vi "CL3IF_GetProgramNo.vi"(8 "error in":errorcluster {"code" format="%x"}, 11 "deviceId":i32) -> (0 "error out":errorcluster {"code" format="%x"}, 2 "programNo":u8)   [LabVIEW 2020, in "Keyence CL-3000.lvlib"]
doc: "This function gets the current program number."
uses:
  Keyence CL-3000.lvlib
  Private/enums/Function Name.ctl
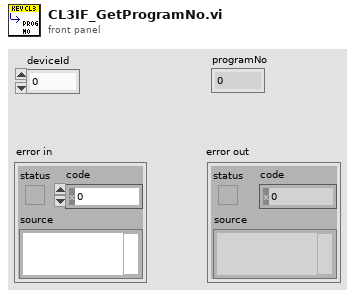
[diagram p1: front panel]
types:
  T1 = typedef "Keyence CL-3000.lvlib/Function Name.ctl" = enum16{"Initialize", "Close", "CL3IF_GetMeasurementData", "CL3IF_GetTrendIndex", "CL3IF_GetTrendData", "CL3IF_GetStorageIndex", "CL3IF_GetStorageData", "CL3IF_AutoZeroMulti", "CL3IF_AutoZeroGroup", "CL3IF_TimingMulti", "CL3IF_TimingGroup", "CL3IF_ResetMulti", "CL3IF_ResetGroup", "CL3IF_LightControl", "CL3IF_MeasurementControl", "CL3IF_SwitchProgram", "CL3IF_GetProgramNo", "CL3IF_StartStorage", "CL3IF_StopStorage", "CL3IF_ClearStorageData", "CL3IF_GetPulseCount", "CL3IF_ResetPulseCount", "CL3IF_GetLightWaveform"}
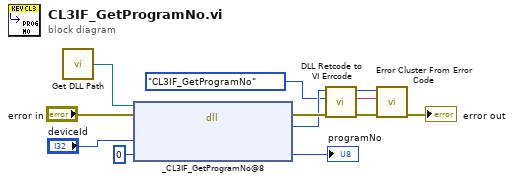
[diagram p0: block diagram]
diagram:
  n1 = call "Get DLL Path.vi"() -> ("DLL Path"=w9:path)  [unwired: 1 in]
  n2 = dll-call lib="C:/Program Files (x86)/National Instruments/LabVIEW 2018/instr.lib/Keyence CL-3000/CL3_IF.dll" fn="_CL3IF_GetProgramNo@8"(path in=w9, error in="error in", "deviceId"="deviceId", "ProgramNo"=u8 0) -> (error out=w7:errorcluster, "RC"=w6:i32, "ProgramNo"=→"programNo":u8)  [unwired: 2 in, 1 out]
  n3 = call "DLL Retcode to VI Errcode.vi"("error in (no error)"=w7, "Function Name"=Function_Name."CL3IF_GetProgramNo", "DLL Retcode"=w6) -> ("error out"=w12:errorcluster, "ErrorMessage"=w4:string, "VI Errcode"=w11:i32)  [unwired: 6 in]
  n4 = call <vilib>:"Error Cluster From Error Code.vi"("error in (no error)"=w12, "error message (\"\")"=w4, "error code (0)"=w11) -> ("error out"=→"error out":errorcluster)  [unwired: 6 in]
